vi "SetUp Wi-Fi Connection.vi"(8 "error in (no error)":errorcluster, 11 "ESP8266 in":refnum<class "ESP8266.lvclass">) -> (0 "error out":errorcluster, 3 "ESP8266 out":refnum<class "ESP8266.lvclass">)   [LabVIEW 2020, in "ESP8266.lvclass"]
uses:
  ESP8266.lvclass
  72a9cd4c-3dee-44fd-92bc-d1c25c4243b1.vi
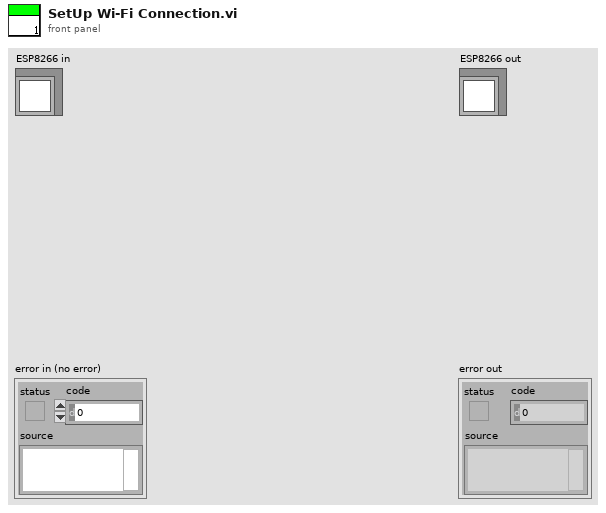
[diagram p1: front panel]
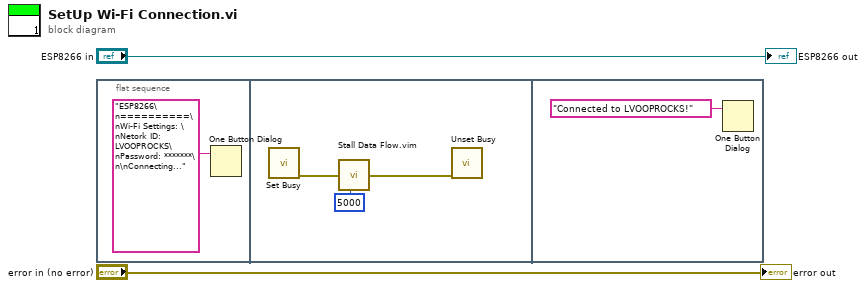
[diagram p0: block diagram]
diagram:
  n1 = flat-sequence {
    frame #0 {
      n2 = One Button Dialog(message="ESP8266\n==========\nWi-Fi Settings: \nNetork ID: LVOOPROCKS\nPassword: *******\n\nConnecting...") -> ()  [unwired: 1 in, 1 out]
    }
    frame #1 {
      n3 = call <vilib>:"Set Busy.vi"() -> ("error out"=w6:errorcluster)  [unwired: 10 in, 1 out]
      n4 = call "Stall Data Flow.vim"("value in"=w6, "milliseconds to wait"=u32 5000) -> ("value out"=w5:errorcluster)  [unwired: 1 out]
      n5 = call <vilib>:"Unset Busy.vi"("error in (no error)"=w5) -> ()  [unwired: 10 in, 1 out]
    }
    frame #2 {
      n6 = One Button Dialog(message="Connected to LVOOPROCKS!") -> ()  [unwired: 1 in, 1 out]
    }
  }
  "error out" <- "error in (no error)"
  "ESP8266 out" <- "ESP8266 in"
